vi "calculate.vi"() -> ()   [LabVIEW 2019]
uses:
  <vilib>/express/express arith-compare/Formula/XNode/ExpressFormulaBlockNode.xnode
panel:
  in  "stop":bool
  out "String":string
  out "output":dbl
  in  "input":dbl
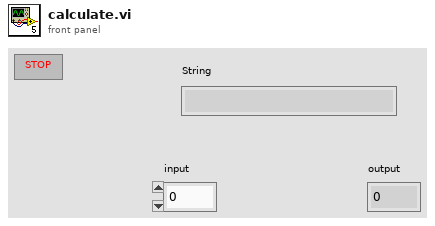
[diagram p1: front panel]
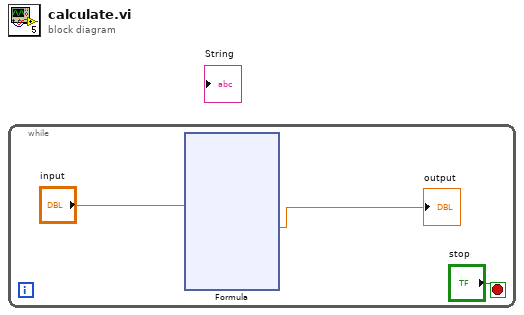
[diagram p0: block diagram]
diagram:
  n1 = while {
    stop <- "stop" stop-if-true
    n2 = xnode "Formula"("X1"="input") -> ("Result"=→"output":dbl)  [unwired: 1 in, 1 out]
  }
